vi "JJMCclase6parte2.vi"() -> ()   [LabVIEW 2011]
panel:
  out "Numeric":dbl
  in  "Detener":bool
  # "Estructura de repeticion"
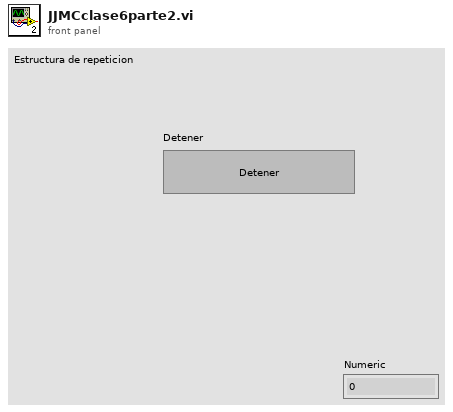
[diagram p1: front panel]
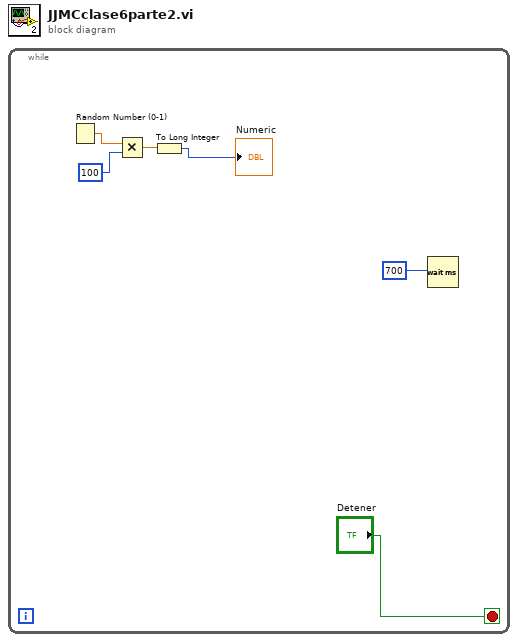
[diagram p0: block diagram]
diagram:
  n1 = while {
    stop <- "Detener" stop-if-true
    n2 = Random Number (0-1)() -> (number: 0 to 1=w5:dbl)
    n3 = Multiply(x=w5, y=100) -> (x*y=w3:dbl)
    n4 = To Long Integer(number=w3) -> (32bit integer=→"Numeric":i32)
    n5 = Wait (ms)(milliseconds to wait=700) -> ()  [unwired: 1 out]
  }
